vi "CleanUp.vi"(0 "object in":refnum<class "MTEC_Async.lvclass">, 5 "error in (no error)":errorcluster) -> (14 "object out":refnum<class "MTEC_Async.lvclass">, 19 "error out":errorcluster)   [LabVIEW 2019, in "MTEC_Async.lvclass"]
uses:
  MTEC_Async.lvclass
  MTEC_Async.lvclass/MTEC_Async.ctl
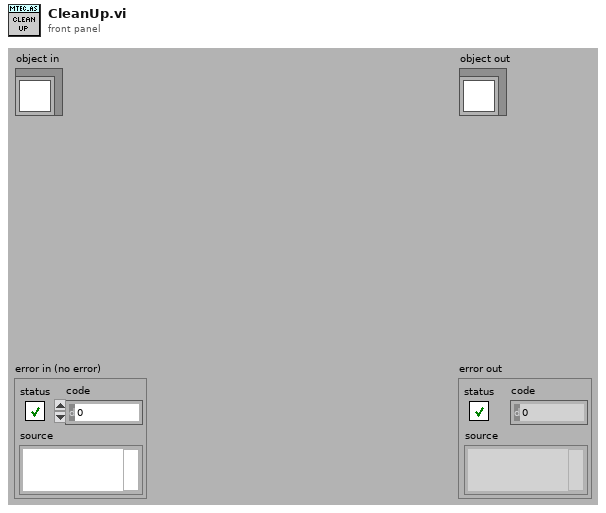
[diagram p1: front panel]
types:
  T1 = cluster{"Message":string, "Message Data":variant}
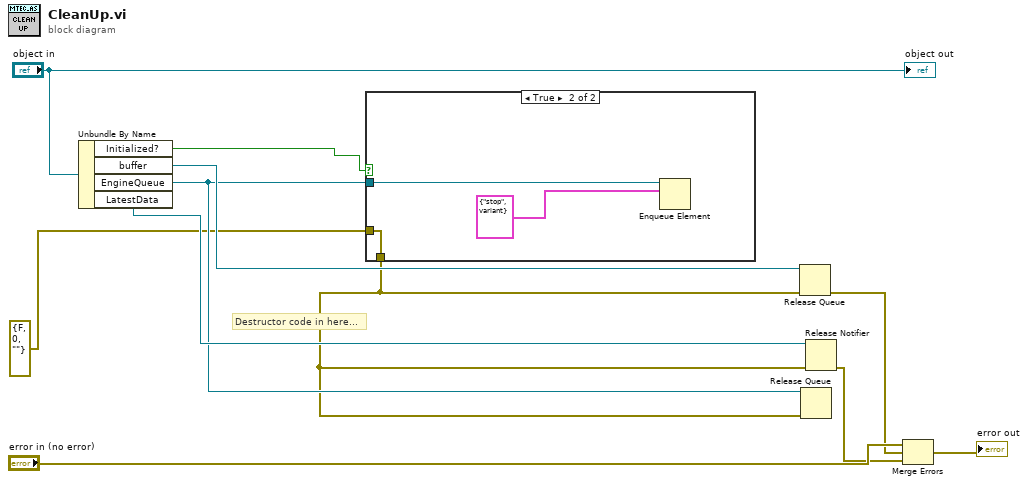
[diagram p0: block diagram]
diagram:
  # "Destructor code in here..."
  n1 = Unbundle By Name("object in") -> ("Initialized?"=w4:bool, "buffer"=w8:refnum<queue>, "EngineQueue"=w3:refnum<queue>, "LatestData"=w5:refnum<notifier>)
  n2 = case shown="True" w4 {
    tunnel: errorcluster {"status"=FALSE, "code"=0, "source"=""} ("error in (no error)") -> [_ w12]
    tunnel: w3 -> [_ w14]
    tunnel: [_ w12] -> w2
    frame False {
    }
    frame True {
      n3 = Enqueue Element(queue=w14, element=T1 {"Message"="stop", "Message Data"=variant}) -> ()  [unwired: 2 in, 3 out]
    }
  }
  n4 = Release Queue(queue=w8, error in (no error)=w2) -> (error out=w7:errorcluster)  [unwired: 1 in, 2 out]
  n5 = Release Queue(queue=w3, error in (no error)=w2) -> ()  [unwired: 1 in, 3 out]
  n6 = Release Notifier(notifier=w5, error in (no error)=w2) -> (error out=w6:errorcluster)  [unwired: 1 in, 2 out]
  n7 = Merge Errors("error in (no error)", w7, w6) -> (→"error out":errorcluster)
  "object out" <- "object in"
